vi "BuildServerRoot.vi"() -> (0 "Server Root":path)   [LabVIEW 2020]
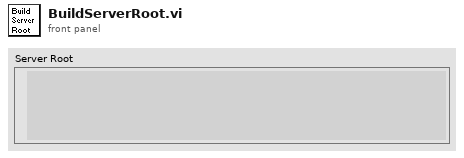
[diagram p1: front panel]
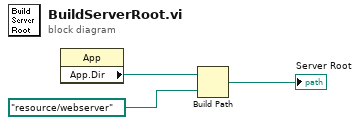
[diagram p0: block diagram]
diagram:
  n1 = property class="App"() -> ("App.Dir"=w3:path)  [unwired: 2 in, 2 out]
  n2 = Build Path(base path=w3, name or relative path=path "resource/webserver") -> (appended path=→"Server Root":path)
